vi "Read Command Responses.vi"(8 "error in (no error)":errorcluster, 11 "Simulado in":refnum<class "Simulado.lvclass">) -> (0 "error out":errorcluster, 2 "Command Responses":variant, 3 "Simulado out":refnum<class "Simulado.lvclass">)   [LabVIEW 2020, in "Simulado.lvclass"]
uses:
  Simulado.lvclass
  Simulado.lvclass/Simulado.ctl
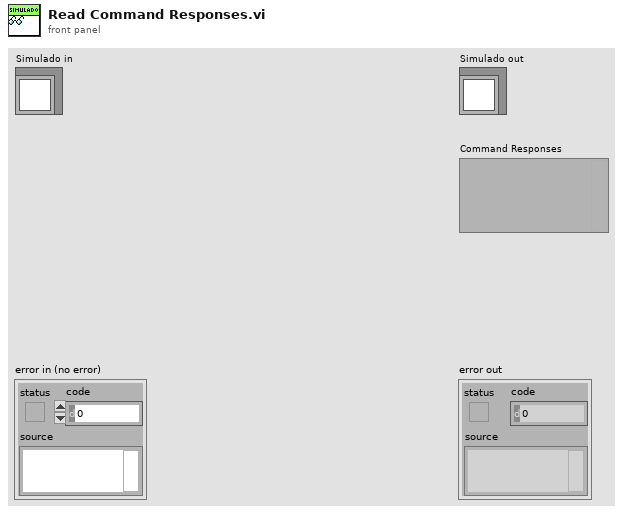
[diagram p1: front panel]
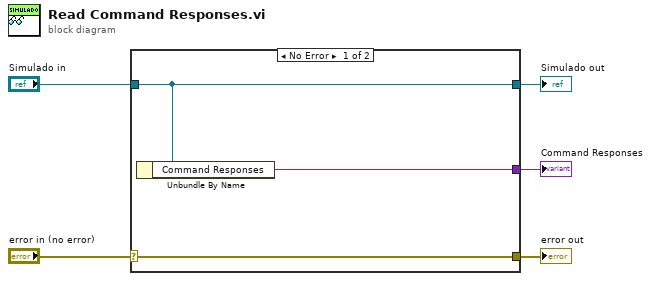
[diagram p0: block diagram]
diagram:
  n1 = case shown="No Error" "error in (no error)" {
    selector: "error in (no error)" -> [w8 w9]
    tunnel: [w8 w9] -> w4
    tunnel: [w7 w10] -> w2
    tunnel: "Simulado in" -> [w7 w10]
    tunnel: [w6 _] -> w1
    frame No Error {
      n2 = Unbundle By Name(w7) -> ("Command Responses"=w6:variant)
    }
    frame Error {
    }
  }
  "error out" <- w4
  "Simulado out" <- w2
  "Command Responses" <- w1
